vi "EnqueueMessage(Poly).vi"   [LabVIEW 2009, in "LapDog.Messaging.v2.lvlib" / "MessageQueue.lvclass"]
uses:
  MessageQueue.lvclass
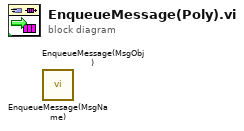
[diagram p0: block diagram]
diagram:
  n1 = call "EnqueueMessage(MsgName).vi"() -> ()  [unwired: 9 in, 3 out]
  n2 = call "EnqueueMessage(MsgObj).vi"() -> ()  [unwired: 9 in, 3 out]
